vi "APT 300XAC Series Perform Test in Program Mode.vi"() -> ()   [LabVIEW 2016]
doc: "Configures the instrument to Program mode and starts the test.\nThe instrument has 50 memory locations with 9 steps for each memory location.\n\nPress stop button to end the test process.\n\n1. Also the Output angle (Start and End) Angle is used as a step parameter in firmware version 2 and system parameter in the firmware version 1.06 respectively.\n\n3. In the firmware version 2.0 and above ,surge drop can be used only in the Program Mode and it is a step parameter.i"
uses:
  Public/Data/Read Test Data (AC Program Mode).vi
  APT 300XAC Series.lvlib
panel:
  out "Test Meter Data Output":T1 {"Timer (s)" format="%.1f"; "Frequency (Hz)" format="%.1f"; "Voltage (V)" format="%.1f"; "RMS Current (A)" format="%.3f"; "Power (W)" format="%.1f"; "Peak Current (A)" format="%.1f"; "Power Factor" format="%.3f"; "Power Resistive (VAR)" format="%.1g"; "Crest Factor" format="%.2f"; "Power Apparent (VA)" format="%.1g"}
  in  "Timeout (10000 ms)":u32=10000
  in  "Starting Step (1)":i32=1
  in  "Enable Over Current Fold Back (F:Disable)":bool
  in  "Start Angle (0)":i32 min=0 max=359
  in  "End Angle: (0)":i32 min=0 max=359
  in  "Frequency High Limit (500 Hz)":dbl=500.0 min=0.0 max=500.0 format="%.1f"
  in  "Frequency Low Limit (40 Hz)":dbl=40.0 min=0.0 max=500.0 format="%.1f"
  in  "Voltage Low Limit (0 V)":dbl min=0.0 max=400.0 format="%.1f"
  in  "Voltage High Limit (300 V)":dbl=300.0 min=0.0 max=400.0 format="%.1f"
  out "Status Byte Register Cluster":T2={"All Pass"=TRUE, "Fail"=FALSE, "Abort"=FALSE, "Test in Process"=FALSE, "Message Available"=FALSE, "Event Summary Bit"=FALSE, "Not Used"=FALSE, "Prompt"=FALSE}
  in  "Stop":bool
  in  "VISA resource name":refnum<visa-resource-name>="COM1"
  in  "Memory Cycle (1)":i32=1 min=0 max=9999 step=1
  in  "Memory (1)":i32=1 min=1 max=50 step=1
  in  "Single Step Mode (F:Disable)":bool
  in  "Loop Cycle (1)":i32=1 min=0 max=9999 step=1
  in  "Step Parameters":T3(array[cluster])=[{"Current High Limit (0 A)"=0.0, "Current Peak High Limit (0 A)"=0.0, "Output AC Voltage (115 V) "=115.0, "Enable Step Connection (F:Disable)"=TRUE, "Step (1)"=1, "Step Cycle (1)"=1, "Power Low Limit (0 W)"=0.0, "Power High Limit (0 W)"=0.0, "Power Factor Low Limit (0)"=0.0, "Power Factor High Limit (0)"=0.0, "Current Low Limit (0 A)"=0.0, "Current Peak Low Limit (0 A)"=0.0, "Dwell (1 s)"=3.0, "Ramp Down Time (0 s)"=2.0, "Delay (0.5 s)"=1.0, "Ramp Up Time (0 s)"=2.0, "Surge Drop Duration (0 ms)"=0.0, "Surge Drop Voltage (100 V) "=100.0, "Surge Drop Start Time (0 ms)"=0.0, "Enable  Continuous Surge Drop (F:Disable)"=FALSE, "Output AC Voltage Frequency (60  Hz)"=60.0, "Voltage Range Mode (1:Auto)"=1, "Enable Surge Drop (F:Disable) "=FALSE, "Step Prompt"={"Enable Prompt"=FALSE, "Prompt ( )"=""}}, {"Current High Limit (0 A)"=0.0, "Current Peak High Limit (0 A)"=8.1387e-320, "Output AC Voltage (115 V) "=110.0, "Enable Step Connection (F:Disable)"=TRUE, "Step (1)"=2, "Step Cycle (1)"=1, "Power Low Limit (0 W)"=0.0, "Power High Limit (0 W)"=0.0, "Power Factor Low Limit (0)"=1.35542481148e-312, "Power Factor High Limit (0)"=0.0, "Current Low Limit (0 A)"=0.0, "Current Peak Low Limit (0 A)"=0.0, "Dwell (1 s)"=15.0, "Ramp Down Time (0 s)"=1.0, "Delay (0.5 s)"=0.5, "Ramp Up Time (0 s)"=1.0, "Surge Drop Duration (0 ms)"=0.0, "Surge Drop Voltage (100 V) "=100.0, "Surge Drop Start Time (0 ms)"=0.0, "Enable  Continuous Surge Drop (F:Disable)"=FALSE, "Output AC Voltage Frequency (60  Hz)"=60.0, "Voltage Range Mode (1:Auto)"=1, "Enable Surge Drop (F:Disable) "=FALSE, "Step Prompt"={"Enable Prompt"=FALSE, "Prompt ( )"=""}}, {"Current High Limit (0 A)"=0.0, "Current Peak High Limit (0 A)"=0.0, "Output AC Voltage (115 V) "=120.0, "Enable Step Connection (F:Disable)"=TRUE, "Step (1)"=3, "Step Cycle (1)"=1, "Power Low Limit (0 W)"=0.0, "Power High Limit (0 W)"=0.0, "Power Factor Low Limit (0)"=0.0, "Power Factor High Limit (0)"=0.0, "Current Low Limit (0 A)"=0.0, "Current Peak Low Limit (0 A)"=0.0, "Dwell (1 s)"=1.0, "Ramp Down Time (0 s)"=0.0, "Delay (0.5 s)"=0.5, "Ramp Up Time (0 s)"=0.0, "Surge Drop Duration (0 ms)"=0.0, "Surge Drop Voltage (100 V) "=100.0, "Surge Drop Start Time (0 ms)"=0.0, "Enable  Continuous Surge Drop (F:Disable)"=FALSE, "Output AC Voltage Frequency (60  Hz)"=65.0, "Voltage Range Mode (1:Auto)"=1, "Enable Surge Drop (F:Disable) "=FALSE, "Step Prompt"={"Enable Prompt"=FALSE, "Prompt ( )"=""}}, {"Current High Limit (0 A)"=0.0, "Current Peak High Limit (0 A)"=0.0, "Output AC Voltage (115 V) "=125.0, "Enable Step Connection (F:Disable)"=FALSE, "Step (1)"=4, "Step Cycle (1)"=1, "Power Low Limit (0 W)"=0.0, "Power High Limit (0 W)"=0.0, "Power Factor Low Limit (0)"=0.0, "Power Factor High Limit (0)"=0.0, "Current Low Limit (0 A)"=0.0, "Current Peak Low Limit (0 A)"=0.0, "Dwell (1 s)"=1.0, "Ramp Down Time (0 s)"=0.0, "Delay (0.5 s)"=0.5, "Ramp Up Time (0 s)"=0.0, "Surge Drop Duration (0 ms)"=0.0, "Surge Drop Voltage (100 V) "=100.0, "Surge Drop Start Time (0 ms)"=0.0, "Enable  Continuous Surge Drop (F:Disable)"=FALSE, "Output AC Voltage Frequency (60  Hz)"=60.0, "Voltage Range Mode (1:Auto)"=1, "Enable Surge Drop (F:Disable) "=FALSE, "Step Prompt"={"Enable Prompt"=FALSE, "Prompt ( )"=""}}] {"Voltage Range Mode (1:Auto)" items=["High", "Auto"]; "Output AC Voltage Frequency (60  Hz)" min=45.0 max=500.0 format="%.1p"; "Surge Drop Start Time (0 ms)" min=0.0 max=99.0; "Surge Drop Voltage (100 V)" min=0.0 max=300.0 format="%#.1f"; "Surge Drop Duration (0 ms)" min=0.0 max=99.0; "Ramp Up Time (0 s)" min=0.0 max=999.9 format="%.1f"; "Delay (0.5 s)" min=0.5 max=999.9 format="%.1f"; "Ramp Down Time (0 s)" min=0.0 max=999.9 format="%.1f"; "Dwell (1 s)" min=0.5 max=999.9 format="%.1f"; "Current Peak Low Limit (0 A)" min=0.0 max=152.0 format="%.3f"; "Current Low Limit (0 A)" min=0.0 max=36.8 format="%.3f"; "Power Factor High Limit (0)" min=0.0 max=1.0 format="%.3f"; "Power Factor Low Limit (0)" min=0.0 max=1.0 format="%.3f"; "Power High Limit (0 W)" min=0.0 max=4000.0 format="%.1f"; "Power Low Limit (0 W)" min=0.0 max=4000.0 format="%.1f"; "Step Cycle (1)" min=0 max=9999 step=1; "Step (1)" min=1 max=9 step=1; "Output AC Voltage (115 V)" min=0.0 max=300.0 format="%.1f"; "Current Peak High Limit (0 A)" min=0.0 max=152.0 format="%.3f"; "Current High Limit (0 A)" min=0.0 max=36.8 format="%.3f"}
  # "APT 300xAC PROGRAM MODE - EXAMPLE"
  # "Note :\n1. Configure the Parameters (Select the instrument VISA resource, voltage etc.,)\n2. Run this VI"
  # "The Step connect mode is used to connect or disconnect one step from another.\nPlease Switch it ON to connect from Step 1 to Step 2."
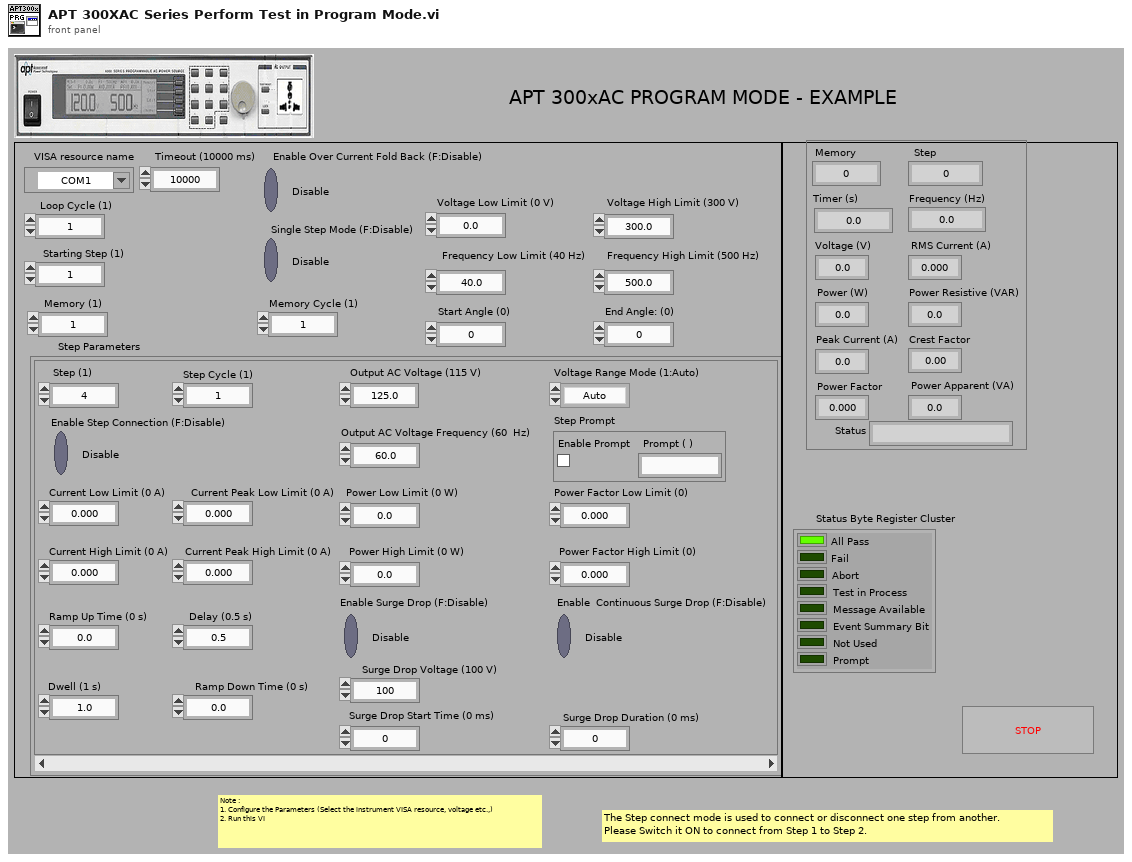
[diagram p1: front panel]
types:
  T1 = cluster{"Memory":i32, "Step":i32, "Timer (s)":dbl, "Frequency (Hz)":dbl, "Voltage (V)":dbl, "RMS Current (A)":dbl, "Power (W)":dbl, "Peak Current (A)":dbl, "Power Factor":dbl, "Status":string, "Power Resistive (VAR)":dbl, "Crest Factor":dbl, "Power Apparent (VA)":dbl}
  T2 = cluster{"All Pass":bool, "Fail":bool, "Abort":bool, "Test in Process":bool, "Message Available":bool, "Event Summary Bit":bool, "Not Used":bool, "Prompt":bool}
  T3 = cluster{"Current High Limit (0 A)":dbl, "Current Peak High Limit (0 A)":dbl, "Output AC Voltage (115 V) ":dbl, "Enable Step Connection (F:Disable)":bool, "Step (1)":i32, "Step Cycle (1)":i32, "Power Low Limit (0 W)":dbl, "Power High Limit (0 W)":dbl, "Power Factor Low Limit (0)":dbl, "Power Factor High Limit (0)":dbl, "Current Low Limit (0 A)":dbl, "Current Peak Low Limit (0 A)":dbl, "Dwell (1 s)":dbl, "Ramp Down Time (0 s)":dbl, "Delay (0.5 s)":dbl, "Ramp Up Time (0 s)":dbl, "Surge Drop Duration (0 ms)":dbl, "Surge Drop Voltage (100 V) ":dbl, "Surge Drop Start Time (0 ms)":dbl, "Enable  Continuous Surge Drop (F:Disable)":bool, "Output AC Voltage Frequency (60  Hz)":dbl, "Voltage Range Mode (1:Auto)":u16, "Enable Surge Drop (F:Disable) ":bool, "Step Prompt":cluster{"Enable Prompt":bool, "Prompt ( )":string}}[]
  T4 = cluster{"Baud Rate":u32, "Parity":u16, "Data Bits":u16, "Stop Bits":u16, "Flow Control":u16}
  T5 = cluster{"Enable Prompt":bool, "Prompt ( )":string}
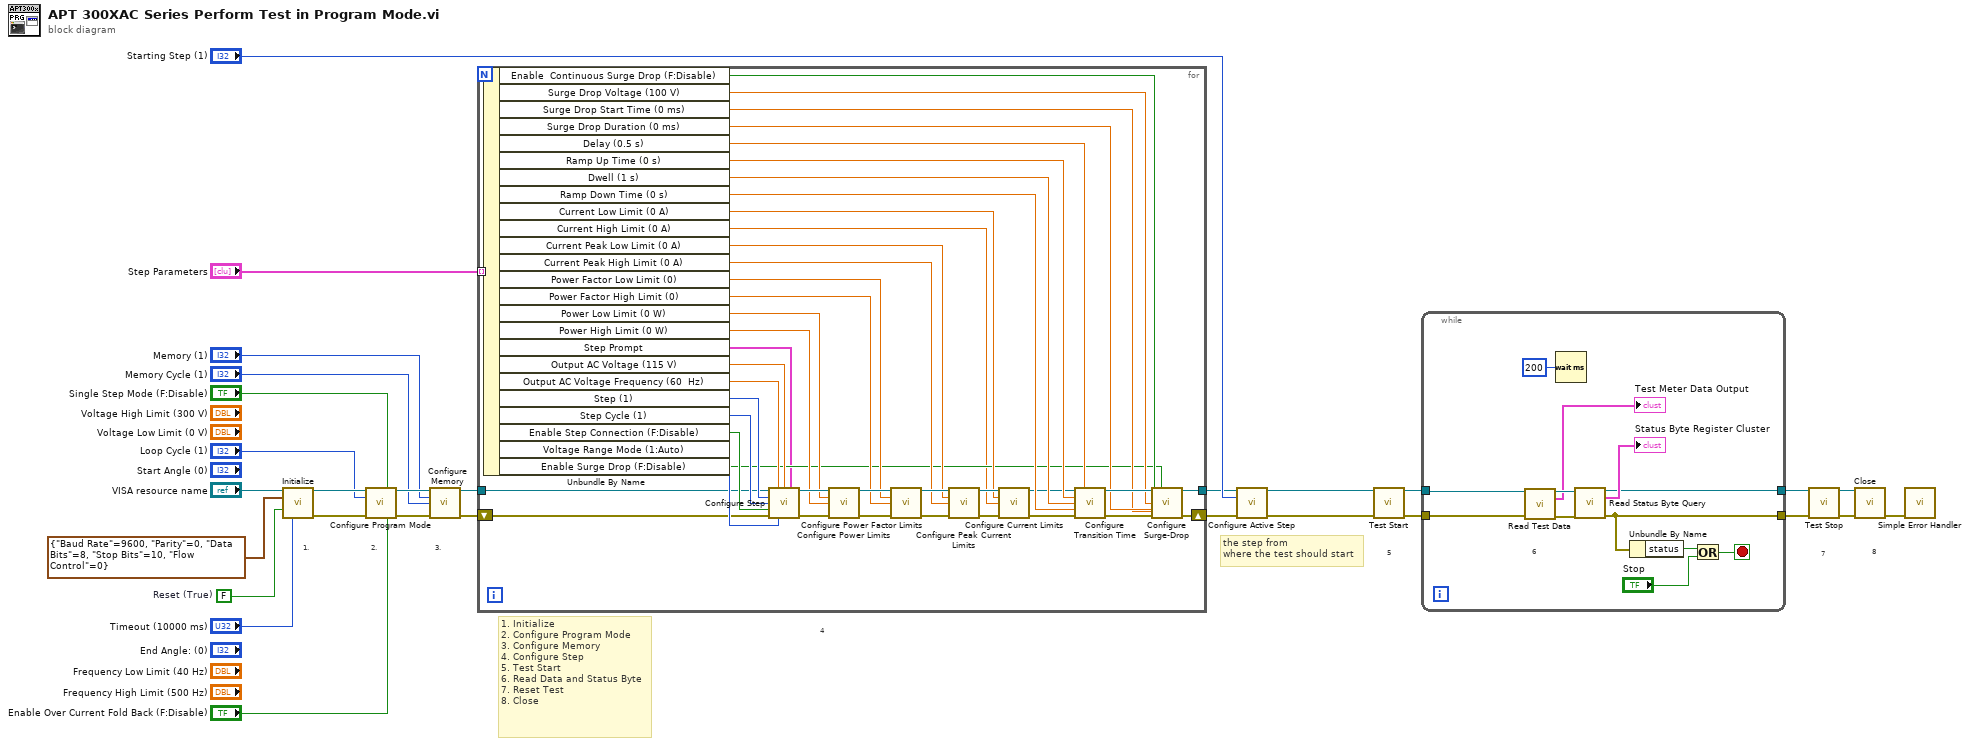
[diagram p0: block diagram]
diagram:
  w26 = FALSE  # Reset (True)
  # "the step from \nwhere the test should start"
  # "5"
  # "4"
  # "1. Initialize\n2. Configure Program Mode\n3. Configure Memory\n4. Configure Step\n5. Test Start\n6. Read Data and Status Byte\n7. Reset Test\n8. Close"
  # "7"
  # "8"
  # "1."
  # "3."
  # "2."
  n1 = call "Initialize.vi"("VISA resource name"="VISA resource name", "Serial Configuration"=T4 {"Baud Rate"=9600, "Parity"=0, "Data Bits"=8, "Stop Bits"=10, "Flow Control"=0}, "Reset (True)"=w26, "Timeout (10000 ms)"="Timeout (10000 ms)") -> ("VISA resource name out"=w25:refnum<visa-resource-name>, "error out"=w27:errorcluster)  [unwired: 10 in]
  n2 = call "Configure Program Mode.vi"("VISA resource name"=w25, "Single Step Mode (F:Disable)"="Single Step Mode (F:Disable)", "Loop Cycle (1)"="Loop Cycle (1)", "error in (no error)"=w27, "Enable Over Current Fold Back (F:Disable)"="Enable Over Current Fold Back (F:Disable)") -> ("VISA resource name out"=w24:refnum<visa-resource-name>, "error out"=w23:errorcluster)  [unwired: 9 in]
  n3 = call "Configure Memory.vi"("VISA resource name"=w24, "Memory (1)"="Memory (1)", "Memory Cycle (1)"="Memory Cycle (1)", "error in (no error)"=w23) -> ("VISA resource name out"=w5:refnum<visa-resource-name>, "error out"=w4:errorcluster)  [unwired: 10 in]
  n4 = for {
    tunnel: "Step Parameters" -> [w67] mode=indexing
    shift-right: [w69] -> w1
    shift-left: w4 -> [w31]
    tunnel: [w68] -> w2
    tunnel: w5 -> [w32]
    n5 = Unbundle By Name(w67) -> ("Enable  Continuous Surge Drop (F:Disable)"=w35:bool, "Surge Drop Voltage (100 V)"=w43:dbl, "Surge Drop Start Time (0 ms)"=w44:dbl, "Surge Drop Duration (0 ms)"=w45:dbl, "Delay (0.5 s)"=w55:dbl, "Ramp Up Time (0 s)"=w54:dbl, "Dwell (1 s)"=w49:dbl, "Ramp Down Time (0 s)"=w48:dbl, "Current Low Limit (0 A)"=w36:dbl, "Current High Limit (0 A)"=w29:dbl, "Current Peak Low Limit (0 A)"=w42:dbl, "Current Peak High Limit (0 A)"=w41:dbl, "Power Factor Low Limit (0)"=w62:dbl, "Power Factor High Limit (0)"=w61:dbl, "Power Low Limit (0 W)"=w60:dbl, "Power High Limit (0 W)"=w59:dbl, "Step Prompt"=w30:T5, "Output AC Voltage (115 V)"=w46:dbl, "Output AC Voltage Frequency (60  Hz)"=w47:dbl, "Step (1)"=w34:i32, "Step Cycle (1)"=w57:i32, "Enable Step Connection (F:Disable)"=w58:bool, "Voltage Range Mode (1:Auto)"=w56:u16, "Enable Surge Drop (F:Disable)"=w33:bool)
    n6 = call "Configure Step.vi"("VISA resource name"=w32, "Output AC Voltage Frequency (60  Hz)"=w47, "Output AC Voltage (115 V)"=w46, "Step Prompt"=w30, "Step (1)"=w34, "Step Cycle (1)"=w57, "Enable Step Connection (F:Disable)"=w58, "error in (no error)"=w31, "Voltage Range Mode (1:Auto)"=w56) -> ("VISA resource name out"=w66:refnum<visa-resource-name>, "error out"=w65:errorcluster)  [unwired: 5 in]
    n7 = call "Configure Power Limits.vi"("VISA resource name"=w66, "Power Low Limit (0 W)"=w60, "Power High Limit (0 W)"=w59, "error in (no error)"=w65) -> ("VISA resource name out"=w64:refnum<visa-resource-name>, "error out"=w63:errorcluster)  [unwired: 10 in]
    n8 = call "Configure Power Factor Limits.vi"("VISA resource name"=w64, "Power Factor Low Limit (0)"=w62, "Power Factor High Limit (0)"=w61, "error in (no error)"=w63) -> ("VISA resource name out"=w53:refnum<visa-resource-name>, "error out"=w52:errorcluster)  [unwired: 10 in]
    n9 = call "Configure Peak Current Limits.vi"("VISA resource name"=w53, "Current Peak Low Limit (0 A)"=w42, "Current Peak High Limit (0 A)"=w41, "error in (no error)"=w52) -> ("VISA resource name out"=w40:refnum<visa-resource-name>, "error out"=w39:errorcluster)  [unwired: 10 in]
    n10 = call "Configure Current Limits.vi"("VISA resource name"=w40, "Current Low Limit (0 A)"=w36, "Current High Limit (0 A)"=w29, "error in (no error)"=w39) -> ("VISA resource name out"=w37:refnum<visa-resource-name>, "error out"=w38:errorcluster)  [unwired: 10 in]
    n11 = call "Configure Transition Time.vi"("VISA resource name"=w37, "Delay (0.5 s)"=w55, "Ramp Up Time (0 s)"=w54, "Dwell (1 s)"=w49, "Ramp Down Time (0 s)"=w48, "error in (no error)"=w38) -> ("VISA resource name out"=w50:refnum<visa-resource-name>, "error out"=w51:errorcluster)  [unwired: 8 in]
    n12 = call "Configure Surge-Drop.vi"("VISA resource name"=w50, "Enable Surge Drop (F:Disable)"=w33, "Enable  Continuous Surge Drop (F:Disable)"=w35, "Surge Drop Voltage (100 V)"=w43, "Surge Drop Duration (0 ms)"=w45, "error in (no error)"=w51, "Surge Drop Start Time (0 ms)"=w44) -> ("VISA resource name out"=w68:refnum<visa-resource-name>, "error out"=w69:errorcluster)  [unwired: 7 in]
  }
  n13 = call "Configure Active Step.vi"("VISA resource name"=w2, "Step (1)"="Starting Step (1)", "error in (no error)"=w1) -> ("VISA resource name out"=w11:refnum<visa-resource-name>, "error out"=w10:errorcluster)  [unwired: 11 in]
  n14 = call "Test Start.vi"("VISA resource name"=w11, "error in (no error)"=w10) -> ("VISA resource name out"=w22:refnum<visa-resource-name>, "error out"=w21:errorcluster)  [unwired: 12 in]
  n15 = while {
    tunnel: [w79] -> w15
    tunnel: [w75] -> w13
    tunnel: w22 -> [w74]
    tunnel: w21 -> [w73]
    stop <- w76 stop-if-true
    # "6"
    n16 = call-poly "Read Test Data.vi"("VISA resource name"=w74, "error in (no error)"=w73) -> ("VISA resource name out"=w72:refnum<visa-resource-name>, "Test Meter Data Output"=→"Test Meter Data Output":T1, "error out"=w71:errorcluster)  [unwired: 11 in]
    n17 = Wait (ms)(milliseconds to wait=u32 200) -> ()  [unwired: 1 out]
    n18 = call "Read Status Byte Query.vi"("VISA resource name"=w72, "error in (no error)"=w71) -> ("VISA resource name out"=w79:refnum<visa-resource-name>, "Status Byte Register"=→"Status Byte Register Cluster":T2, "error out"=w75:errorcluster)  [unwired: 11 in]
    n19 = Unbundle By Name(w75) -> ("status"=w78:bool)
    n20 = Or(x=w78, y="Stop") -> (x .or. y?=w76:bool)
  }
  n21 = call "Test Stop.vi"("VISA resource name"=w15, "error in (no error)"=w13) -> ("VISA resource name out"=w16:refnum<visa-resource-name>, "error out"=w14:errorcluster)  [unwired: 12 in]
  n22 = call "Close.vi"("VISA resource name"=w16, "error in (no error)"=w14) -> ("error out"=w28:errorcluster)  [unwired: 13 in]
  n23 = call <vilib>:"Simple Error Handler.vi"("error in (no error)"=w28) -> ()  [unwired: 4 in, 5 out]
